vi "Tree Column Header.vi"(7 "Action":T1, 10 "Class Name":string, 11 "Tree Ref":refnum<vi>) -> (3 "Tree Column Header":string)   [LabVIEW 2023]
uses:
  controls/action enum.ctl
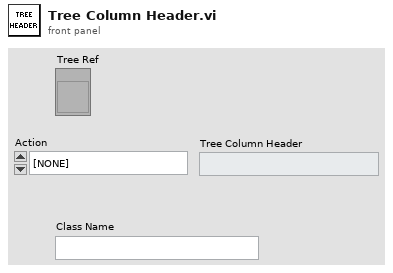
[diagram p1: front panel]
types:
  T1 = typedef "action enum.ctl" = enum16{"[NONE]", "Wire Bundle", "Wire Unbundle", "Terminal Unbundle", "Terminal Bundle", "Bundler Move Up", "Bundler Move Down", "Bundler Insert", "Bundler Remove", "Bundler Remove Unwired", "Bundler Rearrange", "In Place Insert", "In Place Remove", "In Place Remove Unwired", "In Place Rearrange", "Wire Properties", "Wire Method", "Terminal Properties", "Terminal Method", "Property Move Up", "Property Move Down", "Properties Insert", "Properties Remove", "Properties Remove Unwired", "Properties Rearrange", "Method Change", "Class for Constant", "Class For Control", "Class For Node", "Class Name to Clipboard"}
  T2 = enum16{"None", "Cluster", "Property", "Method", "Class"}
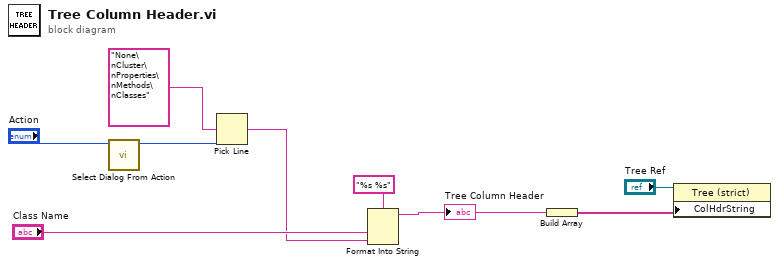
[diagram p0: block diagram]
diagram:
  n1 = call "Select Dialog From Action.vi"("Action"="Action") -> ("Dialog Selection"=w8:T2)  [unwired: 10 in]
  n2 = Pick Line(multi-line string="None\nCluster\nProperties\nMethods\nClasses", line index=w8) -> (output string=w4:string)  [unwired: 1 in]
  n3 = Format Into String(format string="%s %s", "Class Name", w4) -> (resulting string=w2:string)  [unwired: 2 in, 1 out]
  "Tree Column Header" <- w2
  n4 = Build Array(w2) -> (w1:string[])
  n5 = property class="Tree (strict)"(reference="Tree Ref", "ColHdrString"=w1) -> ()  [unwired: 1 in, 2 out]
